vi "AOL Z Cal-Norm coord bypass.vi"(11 "Norm Z":dbl[](array[numeric])) -> (3 "Norm Z":dbl[](array[numeric]))   [LabVIEW 2013]
uses:
  Globals/gl_Calibration globals.vi
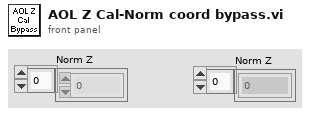
[diagram p1: front panel]
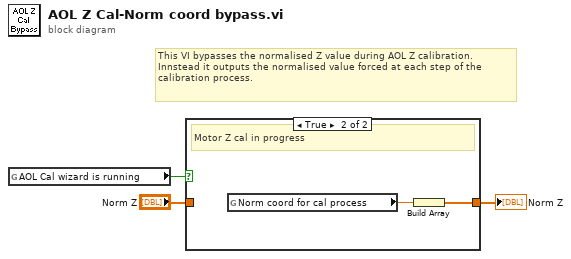
[diagram p0: block diagram]
diagram:
  # "This VI bypasses the normalised Z value during AOL Z calibration.\nInnstead it outputs the normalised value forced at each step of the calibration process."
  n1 = global read "gl_Calibration globals.vi" "AOL Cal wizard is running"() -> (w1:bool)
  n2 = case shown="True" w1 {
    tunnel: [w4 w6] -> w2
    tunnel: "Norm Z" -> [w4 _]
    frame False {
      # "Normal operation"
    }
    frame True {
      # "Motor Z cal in progress"
      n3 = global read "gl_Calibration globals.vi" "Norm coord for cal process"() -> (w5:dbl)
      n4 = Build Array(w5) -> (w6:dbl[])
    }
  }
  "Norm Z" <- w2
